vi "计算长轴xy 长度.vi"(11 "Major Axis":T1) -> (1 "长轴长度":dbl, 2 "第二点x值，y=479":dbl, 3 "第一点x值，y=0":dbl)   [LabVIEW 2015]
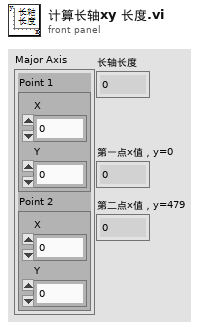
[diagram p1: front panel]
types:
  T1 = cluster{"Point 1":cluster{"X":sgl, "Y":sgl}, "Point 2":cluster{"X":sgl, "Y":sgl}}
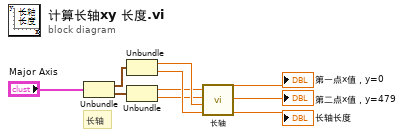
[diagram p0: block diagram]
diagram:
  # "长轴"
  n1 = Unbundle("Major Axis") -> ("Point 1"=w1:cluster{"X":sgl, "Y":sgl}, "Point 2"=w2:cluster{"X":sgl, "Y":sgl})
  n2 = Unbundle(w1) -> ("X"=w5:sgl, "Y"=w8:sgl)
  n3 = Unbundle(w2) -> ("X"=w3:sgl, "Y"=w4:sgl)
  n4 = call "长轴.vi"("y2"=w8, "x2"=w5, "y1"=w4, "x1"=w3) -> ("长轴长度"=→"长轴长度":dbl, "第二点x值，y=479"=→"第二点x值，y=479":dbl, "第一点x值，y=0"=→"第一点x值，y=0":dbl)  [unwired: 5 in]
